vi "Configure Fault Control.vi"(8 "error in (no error)":errorcluster, 9 "NIVS.System Definition Root":refnum<k24>, 10 "VI Reference":refnum<vi>, 11 "Fault Parameters in":T1={"Initialized?"=FALSE, "Label"="", "Default Control Values"=[], "Channel Array"=[], "Fault Control"=[{"String"="", "String 2"="", "String 3"="", "Radio Buttons"=enum."Radio Selection 1"}, {"String"="", "String 2"="", "String 3"="", "Radio Buttons"=enum."Radio Selection 1"}, {"String"="", "String 2"="", "String 3"="", "Radio Buttons"=enum."Radio Selection 1"}, {"String"="", "String 2"="", "String 3"="", "Radio Buttons"=enum."Radio Selection 1"}], "Signals out Array"=[]}) -> (0 "error out":errorcluster, 3 "Fault Parameters out":T1={"Initialized?"=FALSE, "Label"="", "Default Control Values"=[], "Channel Array"=[], "Fault Control"=[{"String"="", "String 2"="", "String 3"="", "Radio Buttons"=enum."Radio Selection 1"}, {"String"="", "String 2"="", "String 3"="", "Radio Buttons"=enum."Radio Selection 1"}, {"String"="", "String 2"="", "String 3"="", "Radio Buttons"=enum."Radio Selection 1"}, {"String"="", "String 2"="", "String 3"="", "Radio Buttons"=enum."Radio Selection 1"}], "Signals out Array"=[]})   [LabVIEW 2013]
doc: "Use this template to create a dialog box with event handling."
uses:
  NationalInstruments.VeriStand.SystemStorage
  Support/Fault Control Parameters.ctl
  NationalInstruments.VeriStand.SystemStorageUI
  <vilib>/NI Veristand/UI Controls/Single Node Browser/NI_VS UI Single Node Browser.lvlib
panel:
  in  "Fault Signals":dbl[](array[numeric])=[0.0, 0.0, 0.0, 0.0, 0.0]
  in  "Channel":refnum<k24>(container)
  in  "Display name (column 1)":u16(ring)
  in  "Make Current Values Default":bool
  in  "Control Label":string
  in  "OK":bool
  in  "Cancel":bool
  # "OK"
  # "OPEN"
  # "GND"
  # "BATT"
  # "COM"
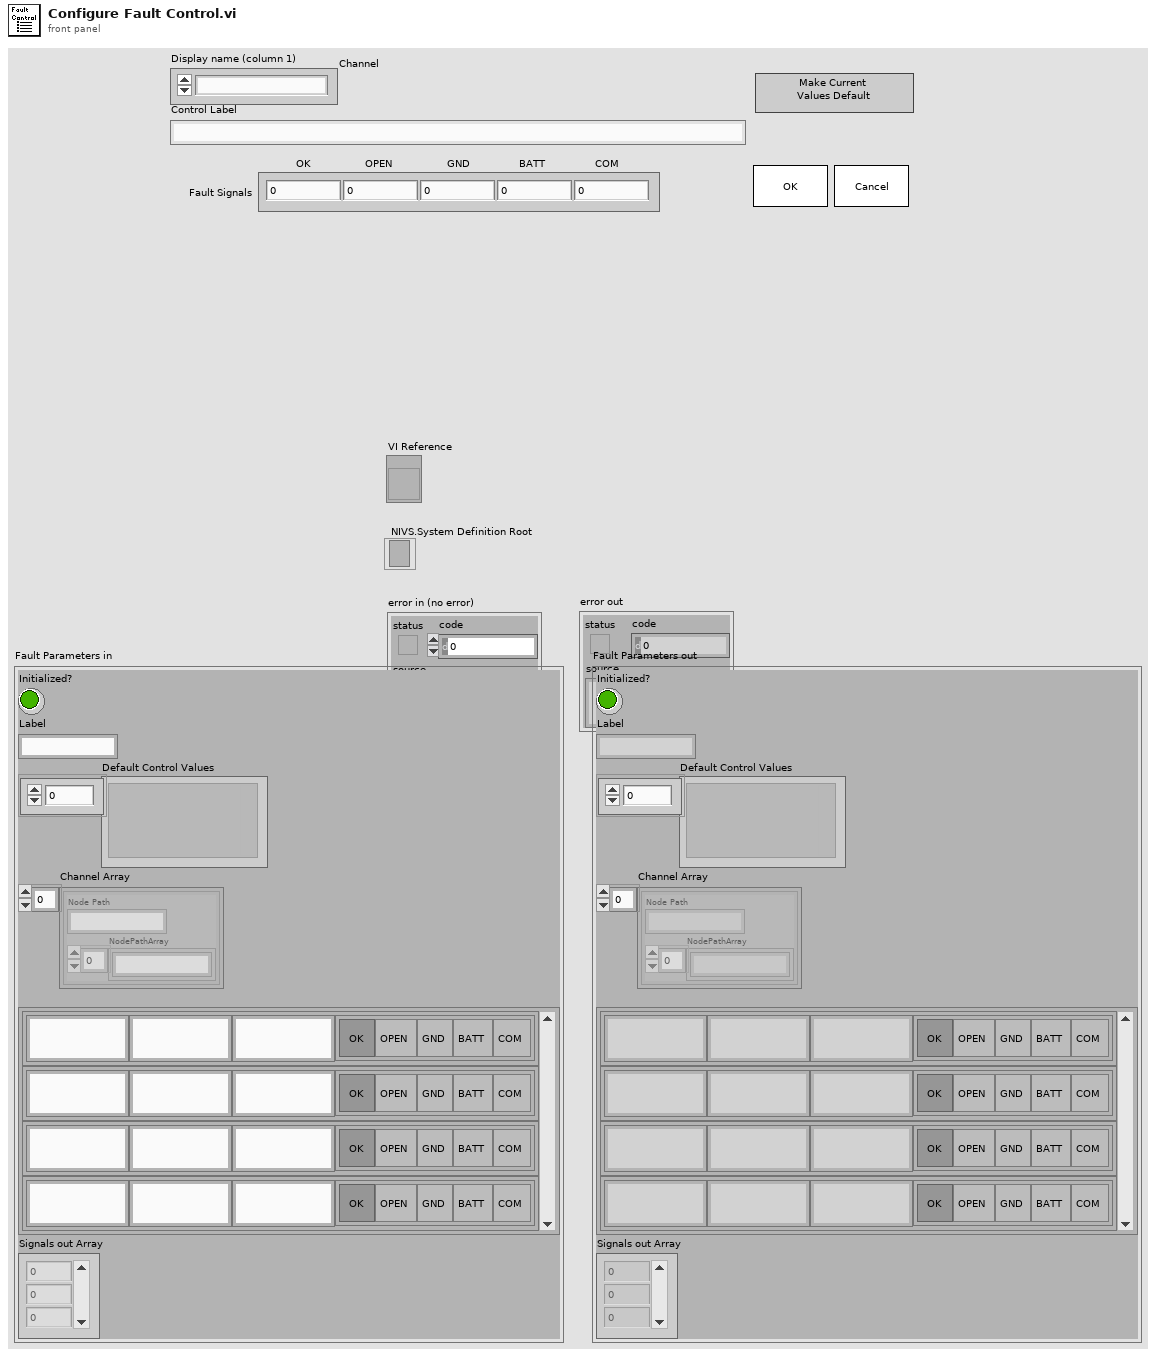
[diagram p1: front panel]
types:
  T1 = typedef "Fault Control Parameters.ctl" = cluster{"Initialized?":bool, "Label":string, "Default Control Values":variant[], "Channel Array":cluster{"NodePathArray":string[], "Node Path":string}[], "Fault Control":cluster{"String":string, "String 2":string, "String 3":string, "Radio Buttons":enum32{"Radio Selection 1", "Radio Selection 2", "Radio Selection 3", "Radio Selection 4", "Radio Selection 5"}}[], "Signals out Array":dbl[]}
  T2 = cluster{"NodePathArray":string[], "Node Path":string}[]
  T3 = cluster{"String":string, "String 2":string, "String 3":string, "Radio Buttons":enum32{"Radio Selection 1", "Radio Selection 2", "Radio Selection 3", "Radio Selection 4", "Radio Selection 5"}}[]
  T4 = cluster{"NodePathArray":string[], "Node Path":string}
  T5 = cluster{"String":string, "String 2":string, "String 3":string, "Radio Buttons":enum32{"Radio Selection 1", "Radio Selection 2", "Radio Selection 3", "Radio Selection 4", "Radio Selection 5"}}
  T6 = typedef "NI_VS UI Single Node Browser.lvlib/Callback Type.ctl" = cluster{"Net Callbacks":refnum<k27>[], "Event":refnum<user-event>}
  T7 = typedef "NI_VS UI Single Node Browser.lvlib/Node Ref.ctl" = refnum<k24>
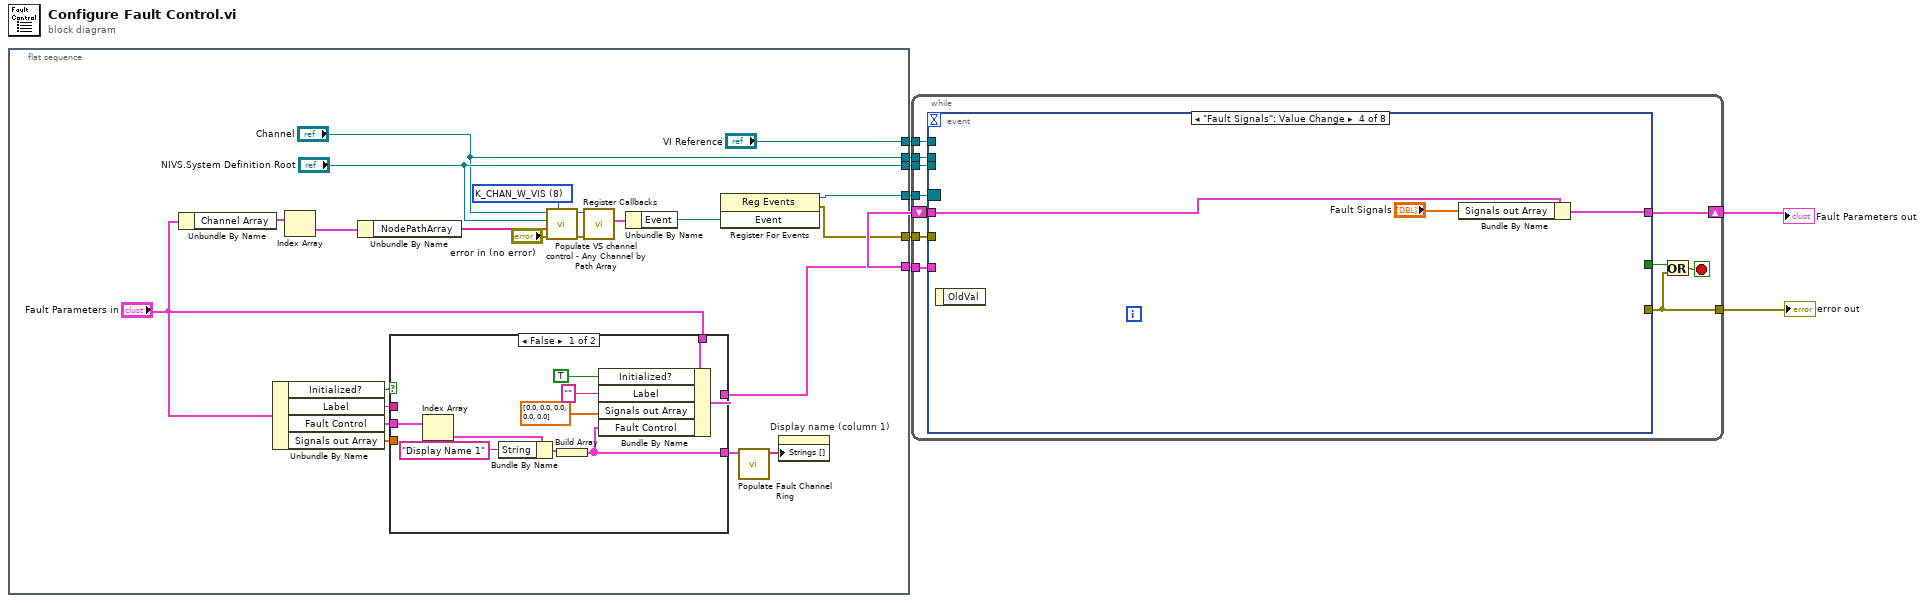
[diagram p0: block diagram]
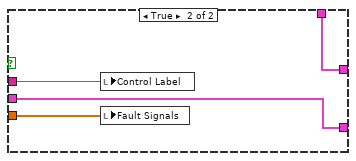
[diagram p2: hidden frame]
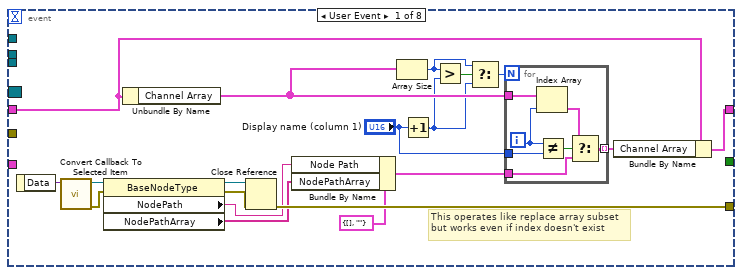
[diagram p3: hidden frame]
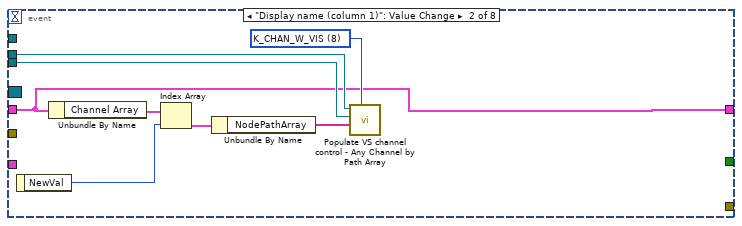
[diagram p4: hidden frame]
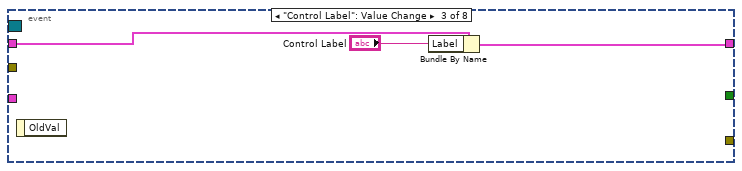
[diagram p5: hidden frame]
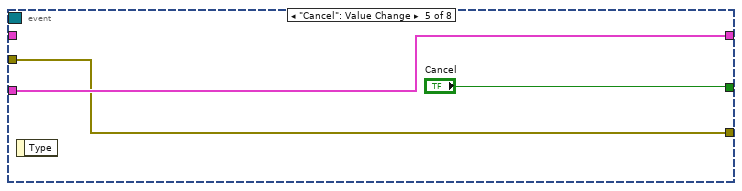
[diagram p6: hidden frame]
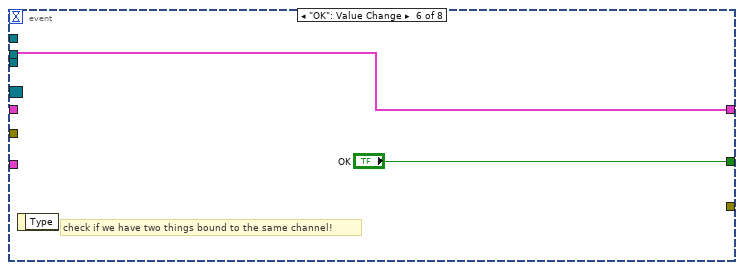
[diagram p7: hidden frame]
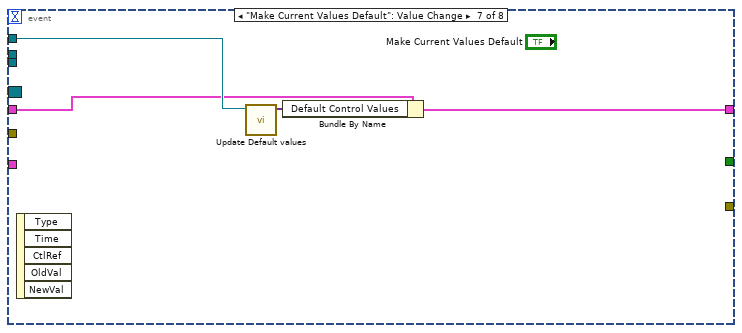
[diagram p8: hidden frame]
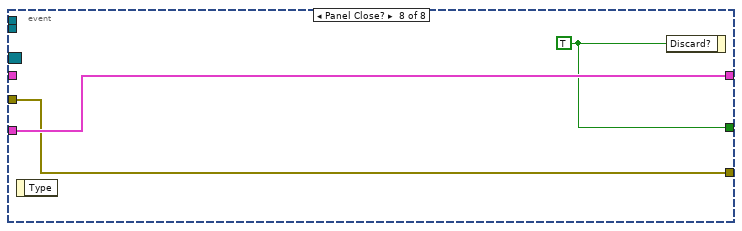
[diagram p9: hidden frame]
diagram:
  n1 = flat-sequence {
    tunnel: ["Channel"] -> w7
    tunnel: ["NIVS.System Definition Root"] -> w6
    tunnel: [w23] -> w5
    tunnel: [w29] -> w3
    tunnel: ["VI Reference"] -> w4
    tunnel: [w22] -> w1
    frame #0 {
      w21 = u8 8 items=["K_CHAN_R", "K_CHAN_W", "K_CHAN_RW", "K_CHAN_VOLT", "K_CHAN_FAULT", "K_ALL", "K_CUSTOM", "K_CHAN_R_VIS", "K_CHAN_W_VIS", "K_CHAN_RW_VIS", "K_CHAN_VOLT_VIS", "K_CHAN_FAULT_VIS"] ("DisplayFilter")
      n2 = Unbundle By Name("Fault Parameters in") -> ("Channel Array"=w17:T2)
      n3 = Unbundle By Name("Fault Parameters in") -> ("Initialized?"=w30:bool, "Label"=w14:string, "Fault Control"=w13:T3, "Signals out Array"=w9:dbl[])
      n4 = Index Array(array=w17) -> (element=w16:T4)  [unwired: 1 in]
      n5 = Unbundle By Name(w16) -> ("NodePathArray"=w15:string[])
      n6 = case shown="False" w30 {
        tunnel: w14 -> [_ w44]
        tunnel: "Fault Parameters in" -> [w40 w43]
        tunnel: [w39 w43] -> w29
        tunnel: w13 -> [w35 w42]
        tunnel: [w31 w42] -> w10
        tunnel: w9 -> [_ w41]
        frame False {
          n7 = Index Array(array=w35) -> (element=w33:T5)  [unwired: 1 in]
          n8 = Bundle By Name(cluster=w33, "String"="Display Name 1") -> (w34:T5)
          n9 = Build Array(w34) -> (w31:T3)
          n10 = Bundle By Name(cluster=w40, "Initialized?"=TRUE ("New?"), "Label"="", "Signals out Array"=dbl[] [0.0, 0.0, 0.0, 0.0, 0.0], "Fault Control"=w31) -> (w39:T1)
        }
        frame True {
          n11 = local write "Control Label"(w44) -> ()
          n12 = local write "Fault Signals"(w41) -> ()
        }
      }
      n13 = call "Populate VS channel control - Any Channel by Path Array.vi"("DisplayFilter"=w21, "error in (no error)"="error in (no error)", "Path Array In"=w15, "NIVS.System Definition Root"="NIVS.System Definition Root", ".NET Refnum in"="Channel") -> ("error out"=w24:errorcluster, ".NET Refnum out"=w25:refnum<k24>)  [unwired: 5 in]
      n14 = call <vilib>:"Register Callbacks.vi"("error in (no error)"=w24, "Single Node Browser"=w25) -> ("Callbacks"=w27:T6)  [unwired: 7 in, 2 out]
      n15 = Unbundle By Name(w27) -> ("Event"=w26:refnum<user-event>)
      n16 = register-events(w26) -> (reference out=w22:refnum<event-registration>, error out=w23:errorcluster)  [unwired: 2 in]
      n17 = call "Populate Fault Channel Ring.vi"("Fault Control"=w10) -> ("Array"=w11:string[])  [unwired: 10 in]
      n18 = property on="Display name (column 1)" class="Ring (strict)"("Strings []"=w11) -> ()  [unwired: 2 in, 2 out]
    }
  }
  n19 = while {
    tunnel: [w46] -> w8
    shift-right: [w52] -> w2
    shift-left: w3 -> [w54]
    tunnel: w3 -> [w53]
    tunnel: w7 -> [w50]
    tunnel: w6 -> [w49]
    tunnel: w5 -> [w48]
    tunnel: w4 -> [w47]
    tunnel: w1 -> [w45]
    stop <- w51 stop-if-true
    n20 = event shown="[3] \"Fault Signals\": Value Change" {
      selector: w45 -> [_ _ _ _ _ _ _ _]
      dyn-events: _ -> [_ _ _ _ _ _ _ _]
      timeout: _ -> [_ _ _ _ _ _ _ _]
      tunnel: [_ _ _ _ "Cancel" "OK" _ w106] -> w55
      tunnel: [w69 _ _ _ w96 _ _ w105] -> w46
      tunnel: w54 -> [w64 w82 w91 w94 _ w100 w102 _]
      tunnel: w53 -> [_ _ _ _ w97 _ _ w107]
      tunnel: [w68 w82 w92 w95 w97 w100 w103 w107] -> w52
      tunnel: w50 -> [_ w85 _ _ _ _ _ _]
      tunnel: w49 -> [_ w84 _ _ _ _ _ _]
      tunnel: w48 -> [_ _ _ _ w96 _ _ w105]
      tunnel: w47 -> [_ _ _ _ _ _ w104 _]
      event User Event {
        # "This operates like replace array subset\nbut works even if index doesn't exist"
        n21 = event-data() -> ("Data"=w70:variant)  [unwired: 1 in]
        n22 = call <vilib>:"Convert Callback To Selected Item.vi"("Data"=w70) -> ("error out"=w71:errorcluster, "Selected Item"=w74:T7)  [unwired: 9 in]
        n23 = property class="BaseNodeType"(reference=w74, error in=w71) -> (reference out=w73:T7, error out=w72:errorcluster, "NodePath"=w66:string, "NodePathArray"=w65:string[])
        n24 = Unbundle By Name(w64) -> ("Channel Array"=w61:T2)
        n25 = Close Reference(reference=w73, error in (no error)=w72) -> (error out=w69:errorcluster)
        n26 = Bundle By Name(cluster=T4 {"NodePathArray"=[], "Node Path"=""} ("Fixed Path"), "Node Path"=w66, "NodePathArray"=w65) -> (w63:T4)
        n27 = Array Size(array=w61) -> (size(s)=w59:i32)
        n28 = Increment(x="Display name (column 1)") -> (x+1=w56:u16)
        n29 = Greater?(x=w59, y=w56) -> (0:w60:bool)
        n30 = Select(t=w59, s=w60, f=w56) -> (s? t:f=w58:i32)
        n31 = for {
          N: w58 -> [_]
          tunnel: "Display name (column 1)" -> [w81]
          tunnel: w63 -> [w79]
          tunnel: w61 -> [w77]
          tunnel: [w78] -> w62 mode=indexing
          i -> [w76]
          n32 = Index Array(array=w77, index=w76) -> (element=w75:T4)
          n33 = Not Equal?(x=w76, y=w81) -> (x != y?=w80:bool)
          n34 = Select(t=w75, s=w80, f=w79) -> (s? t:f=w78:T4)
        }
        n35 = Bundle By Name(cluster=w64, "Channel Array"=w62) -> (w68:T1)
      }
      event "Display name (column 1)": Value Change {
        w83 = u8 8 items=["K_CHAN_R", "K_CHAN_W", "K_CHAN_RW", "K_CHAN_VOLT", "K_CHAN_FAULT", "K_ALL", "K_CUSTOM", "K_CHAN_R_VIS", "K_CHAN_W_VIS", "K_CHAN_RW_VIS", "K_CHAN_VOLT_VIS", "K_CHAN_FAULT_VIS"] ("DisplayFilter")
        n36 = event-data() -> ("NewVal"=w88:u16)  [unwired: 1 in]
        n37 = Unbundle By Name(w82) -> ("Channel Array"=w89:T2)
        n38 = Index Array(array=w89, index=w88) -> (element=w87:T4)
        n39 = Unbundle By Name(w87) -> ("NodePathArray"=w86:string[])
        n40 = call "Populate VS channel control - Any Channel by Path Array.vi"("DisplayFilter"=w83, "Path Array In"=w86, "NIVS.System Definition Root"=w84, ".NET Refnum in"=w85) -> ()  [unwired: 6 in, 2 out]
      }
      event "Control Label": Value Change {
        n41 = event-data() -> ()  [unwired: 1 in, 1 out]
        n42 = Bundle By Name(cluster=w91, "Label"="Control Label") -> (w92:T1)
      }
      event "Fault Signals": Value Change {
        n43 = event-data() -> ()  [unwired: 1 in, 1 out]
        n44 = Bundle By Name(cluster=w94, "Signals out Array"="Fault Signals") -> (w95:T1)
      }
      event "Cancel": Value Change {
        n45 = event-data() -> ()  [unwired: 1 in, 1 out]
      }
      event "OK": Value Change {
        # "check if we have two things bound to the same channel!"
        n46 = event-data() -> ()  [unwired: 1 in, 1 out]
      }
      event "Make Current Values Default": Value Change {
        n47 = event-data() -> ()  [unwired: 1 in, 5 out]
        n48 = call "Update Default values.vi"("VI in"=w104) -> ("Default Values out"=w101:variant[])  [unwired: 10 in]
        n49 = Bundle By Name(cluster=w102, "Default Control Values"=w101) -> (w103:T1)
      }
      event Panel Close? {
        w106 = TRUE ("Cancel")
        n50 = event-data() -> ()  [unwired: 1 in, 1 out]
        n51 = event-data("Discard?"=w106) -> ()  [unwired: 1 in, 1 out]
      }
    }
    n52 = Or(x=w55, y=w46) -> (x .or. y?=w51:bool)
  }
  "error out" <- w8
  "Fault Parameters out" <- w2
